vi "FTW-VAR-Attributes-FindRegexMatches.vi"(8 "error in":errorcluster, 9 "Force Literal Match?":bool, 10 "Regex Match for Attributes":string, 11 "Variant":variant) -> (0 "error out":errorcluster, 1 "Regex Results":cluster{"Match":string, "Submatches":string[]}[](array[cluster]), 2 "Matching Attributes":string[](array[string]), 3 "Variant out":variant)   [LabVIEW 2012]
panel:
  # "Inputs"
  # "Outputs"
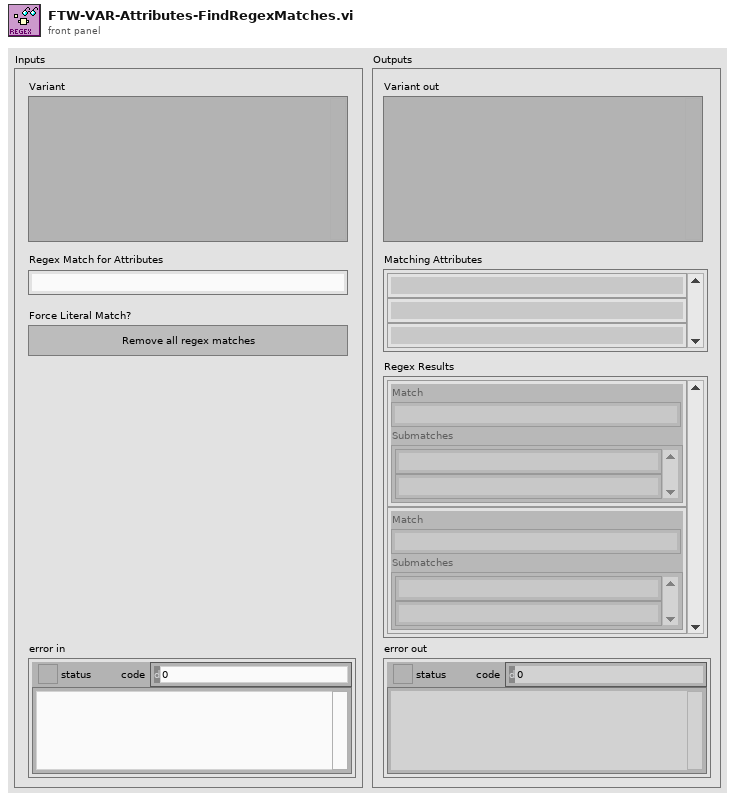
[diagram p1: front panel]
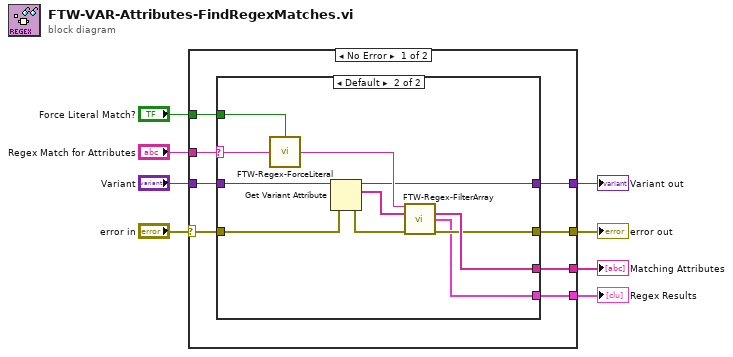
[diagram p0: block diagram]
diagram:
  n1 = case shown="No Error" "error in" {
    selector: "error in" -> [w11 w30]
    tunnel: "Variant" -> [w16 w31]
    tunnel: [w15 w31] -> w7
    tunnel: "Force Literal Match?" -> [w14 _]
    tunnel: [w13 w30] -> w5
    tunnel: "Regex Match for Attributes" -> [w12 _]
    tunnel: [w10 _] -> w2
    tunnel: [w9 _] -> w1
    frame No Error {
      n2 = case shown="Default" w12 {
        selector: w12 -> [_ w25]
        tunnel: w16 -> [w18 w27]
        tunnel: [w18 w21] -> w15
        tunnel: w14 -> [_ w22]
        tunnel: w11 -> [w17 w26]
        tunnel: [w17 w20] -> w13
        tunnel: [_ w24] -> w10
        tunnel: [_ w19] -> w9
        frame "" {
        }
        frame Default {
          n3 = call "FTW-Regex-ForceLiteral.vi"("Input"=w25, "Force Literal Match?"=w22) -> ("Output"=w23:string)
          n4 = Get Variant Attribute(Variant=w27, error in=w26) -> (duplicate Variant=w21:variant, names=w28:string[], error out=w29:errorcluster)  [unwired: 2 in, 1 out]
          n5 = call "FTW-Regex-FilterArray.vi"("Regex Filter"=w23, "Input Array"=w28, "error in"=w29) -> ("Matching Items"=w24:string[], "Regex Results"=w19:cluster{"Match":string, "Submatches":string[]}[], "error out"=w20:errorcluster)  [unwired: 10 in]
        }
      }
    }
    frame Error {
    }
  }
  "error out" <- w5
  "Variant out" <- w7
  "Matching Attributes" <- w2
  "Regex Results" <- w1
